vi "Autonomous Independent.vi"   [LabVIEW 2017]
doc: "This VI is called when autonomous begins, and will automatically be terminated when autonomous ends. You can carry out timed or sensor driven robot movement independently without needing to return to the caller."
uses:
  Public/Documents/Cross The Road Electronics/Phoenix-LabVIEW/Motor Controller/Controls/CTRE_Phoenix_MotorControl_ControlMode.ctl
  <vilib>/Rock Robotics/WPI/Solenoid/WPI_SolenoidValue.ctl
  <vilib>/Rock Robotics/WPI/Utilities/WPI_GetSetVariantRefNum.vi
  <vilib>/Rock Robotics/Network Tables/NT Read String.vi
  <vilib>/Rock Robotics/Network Tables/NT Write Numeric Array.vi
  <vilib>/Rock Robotics/WPI/Ultrasonic/WPI_SonarSRF04DigitalRefNum Registry Get.vi
  Public/Documents/Cross The Road Electronics/Phoenix-LabVIEW/Motor Controller/Get/CTRE_Phoenix_MotorController_GetSelectedSensorData.vi
  <vilib>/Rock Robotics/WPI/Solenoid/WPI_SolenoidSetEnum.vi
  Sling_MN_01/Global 1.vi
panel:
  # "Be sure to right-click and choose Data Operations>>Make Current Value default if you want to save the array values with the VI"
types:
  T1 = typedef "CTRE_Phoenix_MotorControl_ControlMode.ctl" = u16
  T2 = typedef "WPI_JoystickDevRef.ctl" = cluster{"Device":T3}
  T3 = typedef "WPI_JoystickDeviceEnum.ctl" = enum16{"USB 0", "USB 1", "USB 2", "USB 3", "USB 4", "USB 5"}
  T4 = typedef "WPI_GyroDevRef.ctl" = cluster{"DevStatus":errorcluster, "Analog Channel":T5, "Gain (VoltsPerDegree/Second)":dbl, "Gyro Type":enum16{"Analog", "XRS450"}, "Handle":i32, "SPI Bus":T6, "Device Found":bool, "Sample Rate":dbl, "Calibrate On Open":bool, "Offset":dbl}
  T5 = typedef "FPGA_AIChannel.ctl" = enum8{"AI 0", "AI 1", "AI 2", "AI 3", "AI MXP 0", "AI MXP 1", "AI MXP 2", "AI MXP 3", "Invalid"}
  T6 = typedef "spi_bus.ctl" = enum16{"SPI On-Board, CS0", "SPI On-Board, CS1", "SPI On-Board, CS2", "SPI On-Board, CS3", "SPI MXP", "Invalid"}
  T7 = typedef "WPI_MotorControlDeviceRef.ctl" = cluster{"DeviceStatus":errorcluster, "Type":T8, "PWM":cluster{"PWM Channel":T9, "DeadBand":T10}, "CAN":cluster{"Device Number":u8, "SetOutput VI Ref":variant, "GetOutput VI Ref":variant, "Enable VI Ref":variant, "Disable VI Ref":variant, "Data":variant}, "Invert":bool, "DIO PWM":cluster{"PWM \"Enable\" Channel":T9, "DIOChannel":T11, "PWM Rate":dbl}}
  T8 = typedef "WPI_MotorControlType.ctl" = enum16{"PWM", "CAN", "DIO PWM"}
  T9 = typedef "FPGA_DIOPWMChannel.ctl" = enum8{"PWM 0", "PWM 1", "PWM 2", "PWM 3", "PWM 4", "PWM 5", "PWM 6", "PWM 7", "PWM 8", "PWM 9", "PWM MXP 0", "PWM MXP 1", "PWM MXP 2", "PWM MXP 3", "PWM MXP 4", "PWM MXP 5", "PWM MXP 6", "PWM MXP 7", "PWM MXP 8", "PWM MXP 9", "Invalid"}
  T10 = typedef "WPI_PWMDeadband.ctl" = cluster{"Name":string, "maxPositivePwm":i32, "minPositivePwm":i32, "centerPwm":i32, "maxNegativePwm":i32, "minNegativePwm":i32, "angularRange":u16}
  T11 = typedef "FPGA_DIOChannel.ctl" = enum8{"DIO 0", "DIO 1", "DIO 2", "DIO 3", "DIO 4", "DIO 5", "DIO 6", "DIO 7", "DIO 8", "DIO 9", "DIO MXP 0", "DIO MXP 1", "DIO MXP 2", "DIO MXP 3", "DIO MXP 4", "DIO MXP 5", "DIO MXP 6", "DIO MXP 7", "DIO MXP 8", "DIO MXP 9", "DIO MXP 10", "DIO MXP 11", "DIO MXP 12", "DIO MXP 13", "DIO MXP 14", "DIO MXP 15", "SPI Port CS1", "SPI Port CS2", "SPI Port CS3", "SPI Port MISO", "SPI Port MOSI", "Invalid"}
  T12 = typedef "WPI_UltrasonicDeviceRef.ctl" = cluster{"DevStatus":errorcluster, "Ping Channel":T11, "Echo Channel":T11, "CntIndex":T13}
  T13 = typedef "FPGA_CounterCtrSystemIndex.ctl" = enum8{"Ctr 0", "Ctr 1", "Ctr 2", "Ctr 3", "Ctr 4", "Ctr 5", "Ctr 6", "Ctr 7", "Invalid"}
  T14 = typedef "WPI_SolenoidDevRef.ctl" = cluster{"DevStatus":errorcluster, "Pneumatics Control Module":u8, "Forward Solenoid Channel":T15, "Reverse Solenoid Channel":T15}
  T15 = typedef "WPI_SolenoidChannel.ctl" = enum8{"Solenoid 0", "Solenoid 1", "Solenoid 2", "Solenoid 3", "Solenoid 4", "Solenoid 5", "Solenoid 6", "Solenoid 7", "Invalid"}
  T16 = typedef "WPI_SolenoidValue.ctl" = enum16{"Off", "On", "Forward", "Reverse"}
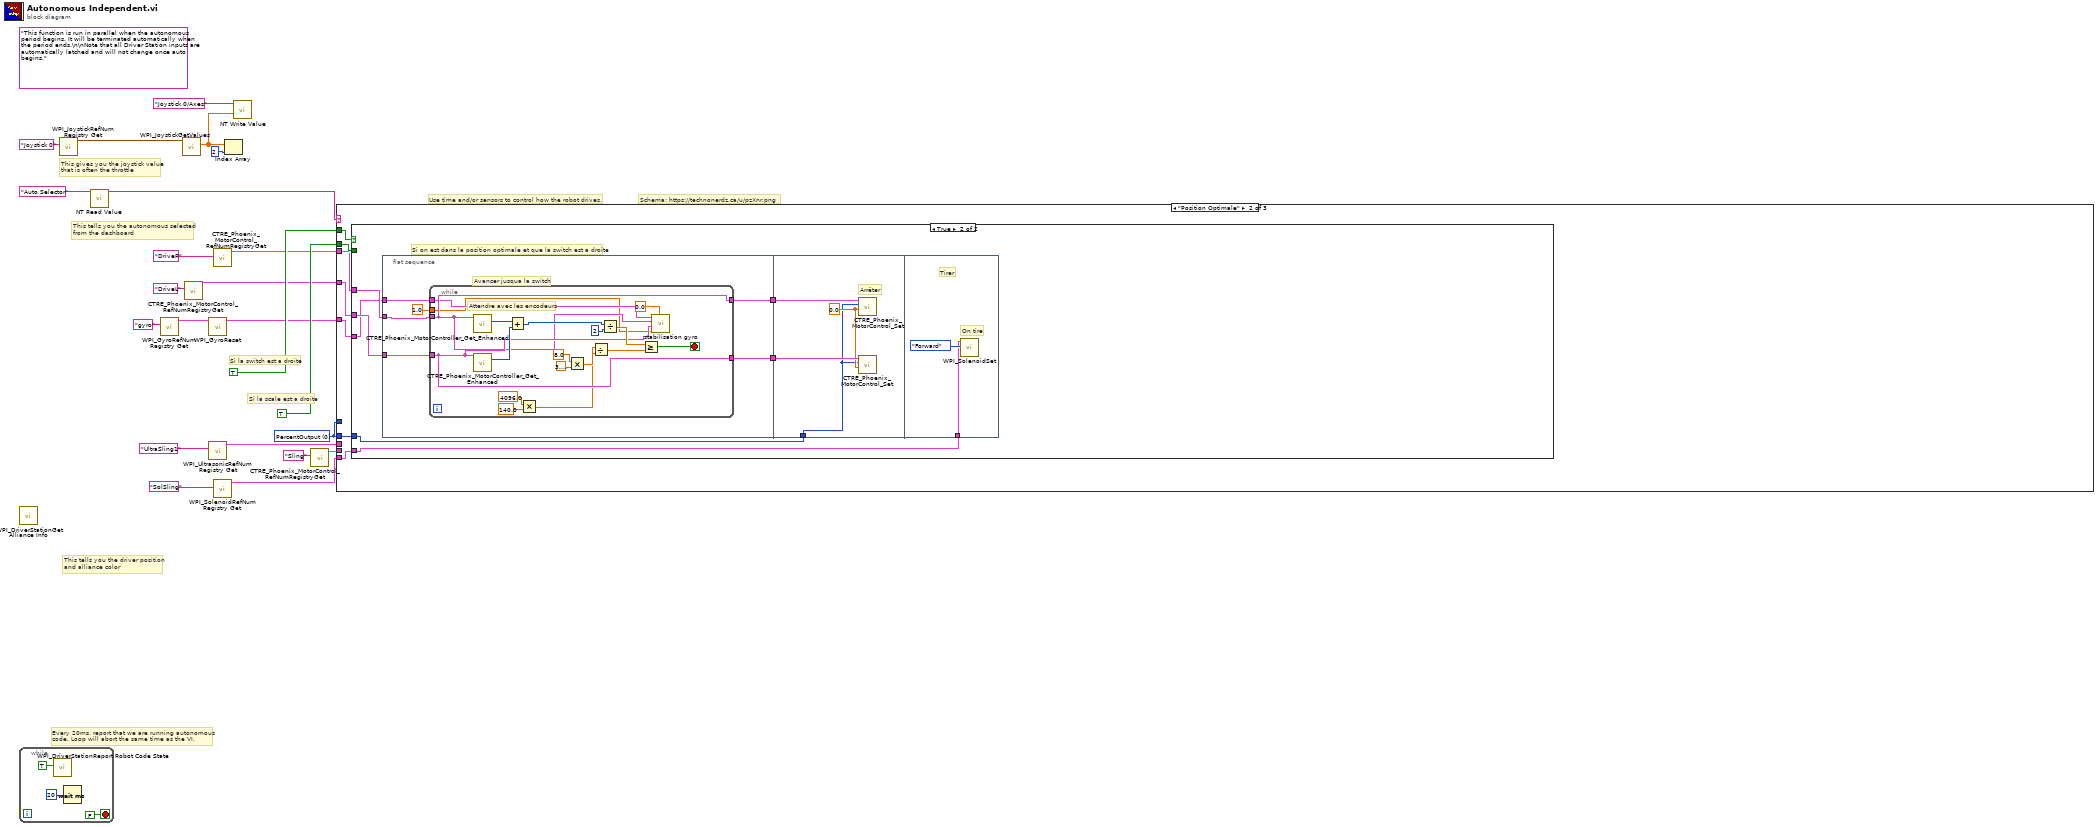
[diagram p0: block diagram]
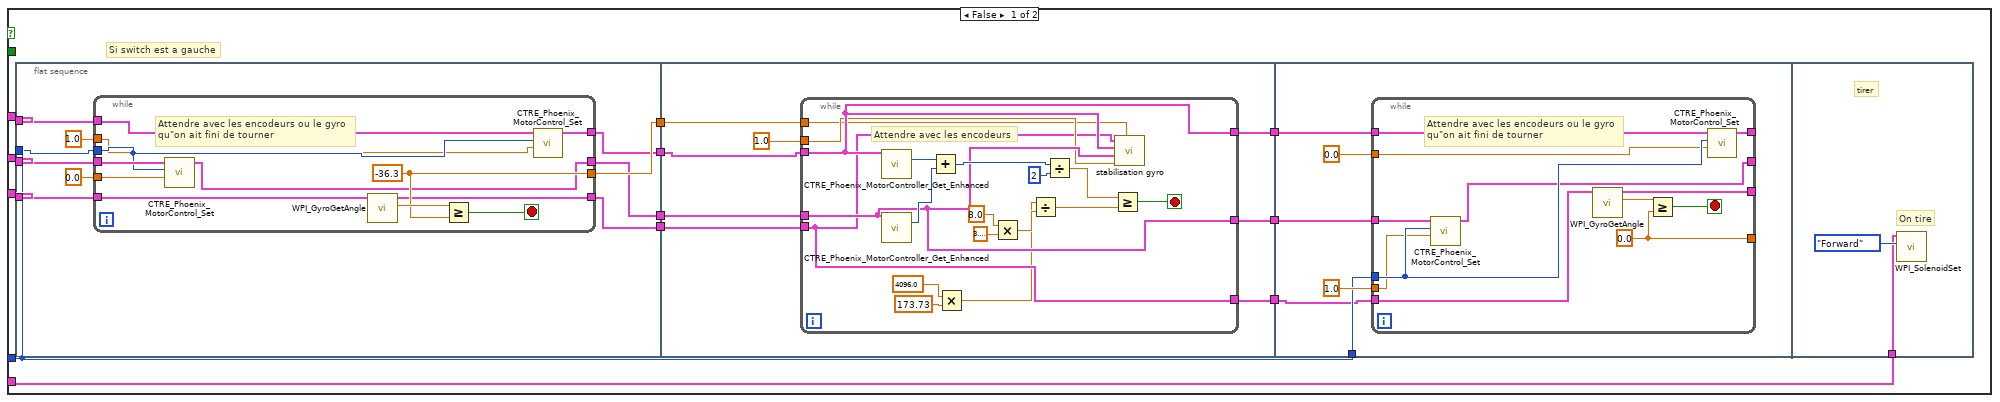
[diagram p3: hidden frame]
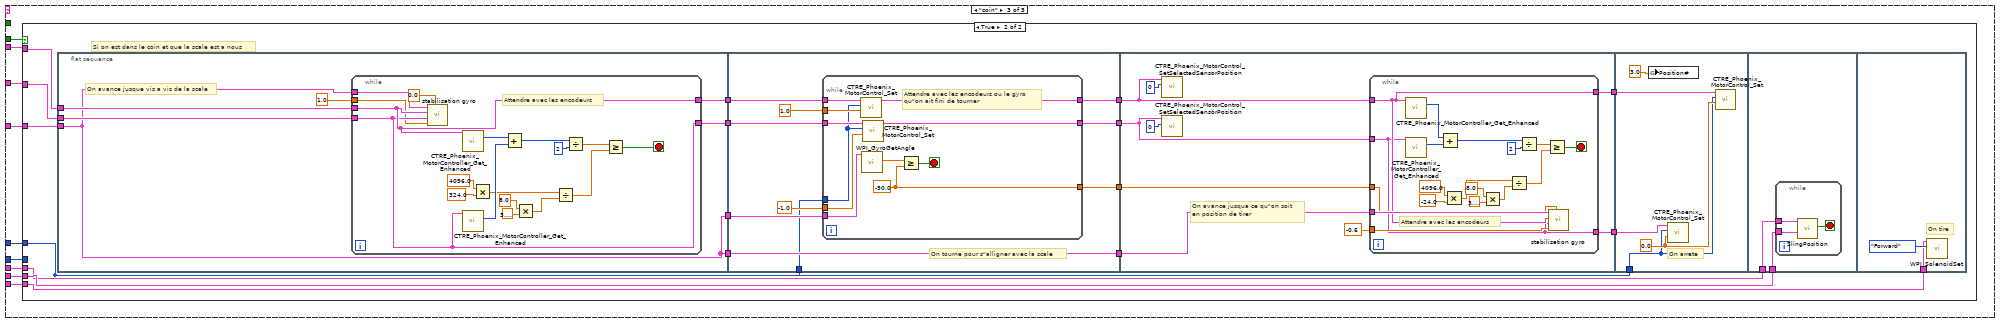
[diagram p4: hidden frame]
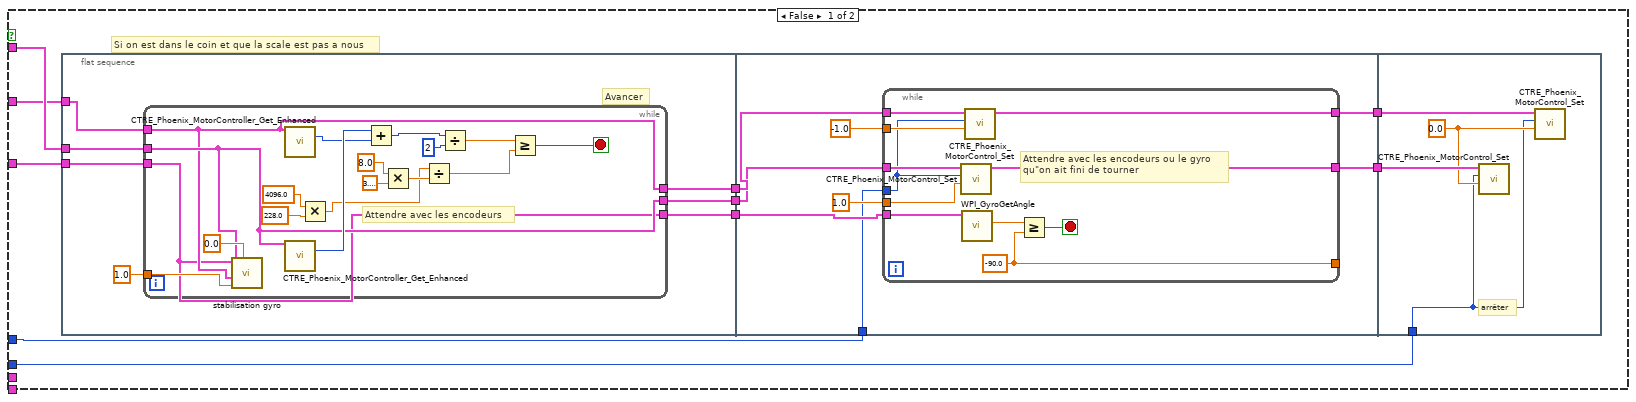
[diagram p5: hidden frame]
diagram:
  w7 = T1 0 items=["PercentOutput"=0, "Position"=1, "Velocity"=2, "Current"=3, "Follower"=5, "MotionProfile"=6, "MotionMagic"=7, "MotionMagicArc"=8, "MotionProfileArc"=10, "Disabled"=15] ("Control Mode")
  (unwired) "This function is run in parallel when the autonomous period begins. It will be terminated automatically when the period ends.\n\nNote that all Driver Station inputs are automatically latched and will not change once auto begins."
  # "Schema: https://technonerdz.ca/u/pzXnr.png"
  # "Si la switch est a droite"
  # "Si la scale est a droite"
  # "This tells you the autonomous selected\nfrom the dashboard"
  # "Every 20ms, report that we are running autonomous\ncode. Loop will abort the same time as the VI."
  # "This gives you the joystick value\nthat is often the throttle"
  # "Use time and/or sensors to control how the robot drives."
  # "This tells you the driver position\nand alliance color"
  n1 = call <vilib>:"WPI_DriverStationGet Alliance Info.vi"() -> ()  [unwired: 12 out]
  n2 = while {
    stop <- FALSE stop-if-true
    n3 = call <vilib>:"WPI_DriverStationReport Robot Code State.vi"("Autonomous"=TRUE) -> ()  [unwired: 10 in, 1 out]
    n4 = Wait (ms)(milliseconds to wait=u32 20) -> ()  [unwired: 1 out]
  }
  n5 = call <vilib>:"WPI_JoystickRefNum Registry Get.vi"("refnum name"="Joystick 0") -> ("JoystickDevRef"=w22:T2)  [unwired: 1 in, 9 out]
  n6 = call-poly <vilib>:"NT Read Value.vi"("Name"="Auto Selector") -> ("String"=w19:string)  [unwired: 9 in, 1 out]
  n7 = call <vilib>:"WPI_GyroRefNum Registry Get.vi"("refnum name"="gyro") -> ("GyroDevRef"=w9:T4)  [unwired: 9 in, 1 out]
  n8 = call <vilib>:"WPI_JoystickGetValues.vi"("JoystickDevRef"=w22) -> ("Axes"=w18:dbl[])  [unwired: 6 in, 4 out]
  n9 = call "CTRE_Phoenix_MotorControl_RefNumRegistryGet.vi"("refnum name"="DriveL") -> ("PhoenixMotorControlDevRef"=w11:T7)  [unwired: 9 in, 1 out]
  n10 = call <vilib>:"WPI_GyroReset.vi"("GyroDevRef"=w9) -> ("GyroDevRef"=w8:T4)  [unwired: 9 in, 1 out]
  n11 = call-poly <vilib>:"WPI_UltrasonicRefNum Registry Get.vi"("refnum name"="UltraSling1") -> ("SonarSRF04DevRef"=w1:T12)  [unwired: 9 in, 1 out]
  n12 = call "CTRE_Phoenix_MotorControl_RefNumRegistryGet.vi"("refnum name"="DriveR") -> ("PhoenixMotorControlDevRef"=w12:T7)  [unwired: 9 in, 1 out]
  n13 = call <vilib>:"WPI_SolenoidRefNum Registry Get.vi"("refnum name"="SolSling") -> ("SolenoidDevRef"=w5:T14)  [unwired: 9 in, 1 out]
  n14 = Index Array(array=w18, index=2) -> ()  [unwired: 1 out]
  n15 = call-poly <vilib>:"NT Write Value.vi"("Numeric Array"=w18, "Name"="Joystick 0/Axes") -> ()  [unwired: 9 in, 1 out]
  n16 = call "CTRE_Phoenix_MotorControl_RefNumRegistryGet.vi"("refnum name"="Sling") -> ("PhoenixMotorControlDevRef"=w2:T7)  [unwired: 9 in, 1 out]
  n17 = case shown="\"Position Optimale\"" w19 {
    tunnel: TRUE -> [_ w32 w159]
    tunnel: TRUE -> [_ w33 _]
    tunnel: w12 -> [_ w31 w158]
    tunnel: w11 -> [_ w30 w157]
    tunnel: w8 -> [_ w29 w156]
    tunnel: w7 -> [_ _ w155]
    tunnel: w7 -> [_ w28 w154]
    tunnel: w5 -> [_ w27 w153]
    tunnel: w2 -> [_ _ w152]
    tunnel: w1 -> [_ _ w151]
    frame Default {
      # "You can put your main auto here, or you can right-click on the case and make any\nother frame be the default case."
      # "This is the frame that will execute if no selection is made, or if it is not recognized"
    }
    frame "Position Optimale" {
      n18 = case shown="True" w33 {
        tunnel: w32 -> [_ _]
        tunnel: w31 -> [w45 w120]
        tunnel: w30 -> [w44 w119]
        tunnel: w29 -> [w43 w116]
        tunnel: w28 -> [w38 w115]
        tunnel: w27 -> [w34 w114]
        frame False {
          # "Si switch est a gauche"
          n19 = flat-sequence {
            tunnel: w45 -> [w55]
            tunnel: w44 -> [w54]
            tunnel: w38 -> [w53]
            tunnel: w43 -> [w50]
            tunnel: [w49] -> w42
            tunnel: [w48] -> w41
            tunnel: [w47] -> w40
            tunnel: [w46] -> w39
            tunnel: w42 -> [w74]
            tunnel: w41 -> [w73]
            tunnel: w40 -> [w72]
            tunnel: w39 -> [w71]
            tunnel: [w70] -> w37
            tunnel: [w69] -> w36
            tunnel: [w68] -> w35
            tunnel: w38 -> [w97]
            tunnel: w37 -> [w96]
            tunnel: w36 -> [w95]
            tunnel: w35 -> [w94]
            tunnel: w34 -> [w112]
            frame #0 {
              n20 = while {
                tunnel: w55 -> [w66]
                tunnel: w54 -> [w65]
                tunnel: w53 -> [w64]
                tunnel: 1.0 ("right") -> [w63]
                tunnel: 0.0 ("left") -> [w62]
                tunnel: w50 -> [w61]
                tunnel: [w59] -> w49
                tunnel: [w58] -> w48
                tunnel: [w57] -> w47
                tunnel: [w56] -> w46
                stop <- w60 stop-if-true
                w59 = -36.3 ("y")
                # "Attendre avec les encodeurs ou le gyro\nqu\"on ait fini de tourner"
                n21 = call "CTRE_Phoenix_MotorControl_Set.vi"("Output"=w62, "Control Mode"=w64, "PhoenixMotorControlDevRef"=w65) -> ("PhoenixMotorControlDevRef"=w58:T7)  [unwired: 7 in, 1 out]
                n22 = call <vilib>:"WPI_GyroGetAngle.vi"("GyroDevRef"=w61) -> ("Angle"=w67:dbl, "GyroDevRef"=w56:T4)  [unwired: 6 in, 3 out]
                n23 = Greater Or Equal?(x=w67, y=w59) -> (x >= y?=w60:bool)
                n24 = call "CTRE_Phoenix_MotorControl_Set.vi"("Output"=w63, "Control Mode"=w64, "PhoenixMotorControlDevRef"=w66) -> ("PhoenixMotorControlDevRef"=w57:T7)  [unwired: 7 in, 1 out]
              }
            }
            frame #1 {
              n25 = while {
                tunnel: 1.0 ("right") -> [w85]
                tunnel: w72 -> [w87]
                tunnel: w73 -> [w86]
                tunnel: [w87] -> w70
                tunnel: [w86] -> w69
                tunnel: [w83] -> w68
                tunnel: w74 -> [w84]
                tunnel: w71 -> [w83]
                stop <- w88 stop-if-true
                # "Attendre avec les encodeurs"
                n26 = call-poly "CTRE_Phoenix_MotorController_Get_Enhanced.vi"("PhoenixMotorControlDevRef"=w87) -> ("Position (Raw Sensor Units)"=w93:i32)  [unwired: 11 in, 3 out]
                n27 = call-poly "CTRE_Phoenix_MotorController_Get_Enhanced.vi"("PhoenixMotorControlDevRef"=w86) -> ("Position (Raw Sensor Units)"=w92:i32)  [unwired: 11 in, 3 out]
                n28 = Add(x=w93, y=w92) -> (x+y=w91:i32)
                n29 = Multiply(x=4096.0, y=173.73) -> (x*y=w81:dbl)
                n30 = Multiply(x=8.0, y=3.141592653589793) -> (x*y=w82:dbl)
                n31 = Divide(x=w81, y=w82) -> (x/y=w76:dbl)
                n32 = Divide(x=w91, y=2) -> (x/y=w89:dbl)
                n33 = Greater Or Equal?(x=w89, y=w76) -> (x >= y?=w88:bool)
                n34 = call "stabilisation gyro.vi"("Direction degres"=w84, "speed"=w85, "LeftMotorDevRef"=w86, "RightMotorDevRef"=w87, "gyroDevRef"=w83) -> ()  [unwired: 7 in]
              }
            }
            frame #2 {
              n35 = while {
                tunnel: w96 -> [w110]
                tunnel: w95 -> [w109]
                tunnel: w97 -> [w108]
                tunnel: 0.0 ("right") -> [w107]
                tunnel: 1.0 ("left") -> [w106]
                tunnel: w94 -> [w105]
                tunnel: [w103] -> _
                tunnel: [w102] -> _
                tunnel: [w101] -> _
                tunnel: [w100] -> _
                stop <- w104 stop-if-true
                w103 = 0.0 ("y")
                # "Attendre avec les encodeurs ou le gyro\nqu\"on ait fini de tourner"
                n36 = call "CTRE_Phoenix_MotorControl_Set.vi"("Output"=w106, "Control Mode"=w108, "PhoenixMotorControlDevRef"=w109) -> ("PhoenixMotorControlDevRef"=w102:T7)  [unwired: 7 in, 1 out]
                n37 = call <vilib>:"WPI_GyroGetAngle.vi"("GyroDevRef"=w105) -> ("Angle"=w111:dbl, "GyroDevRef"=w100:T4)  [unwired: 6 in, 3 out]
                n38 = Greater Or Equal?(x=w111, y=w103) -> (x >= y?=w104:bool)
                n39 = call "CTRE_Phoenix_MotorControl_Set.vi"("Output"=w107, "Control Mode"=w108, "PhoenixMotorControlDevRef"=w110) -> ("PhoenixMotorControlDevRef"=w101:T7)  [unwired: 7 in, 1 out]
              }
            }
            frame #3 {
              # "On tire"
              # "tirer"
              n40 = call-poly <vilib>:"WPI_SolenoidSet.vi"("Value"=WPI_SolenoidValue."Forward", "SolenoidDevRef"=w112) -> ()  [unwired: 8 in, 2 out]
            }
          }
        }
        frame True {
          # "Si on est dans la position optimale et que la switch est a droite"
          n41 = flat-sequence {
            tunnel: w120 -> [w125]
            tunnel: w119 -> [w124]
            tunnel: [w123] -> w118
            tunnel: [w122] -> w117
            tunnel: w116 -> [w121]
            tunnel: w118 -> [w148]
            tunnel: w117 -> [w147]
            tunnel: w115 -> [w145]
            tunnel: w114 -> [w149]
            frame #0 {
              # "Avancer jusqua la switch"
              n42 = while {
                tunnel: 1.0 ("right") -> [w134]
                tunnel: w125 -> [w137]
                tunnel: w124 -> [w138]
                tunnel: [w138] -> w123
                tunnel: [w137] -> w122
                tunnel: w121 -> [w136]
                stop <- w139 stop-if-true
                # "Attendre avec les encodeurs"
                n43 = call-poly "CTRE_Phoenix_MotorController_Get_Enhanced.vi"("PhoenixMotorControlDevRef"=w137) -> ("Position (Raw Sensor Units)"=w144:i32)  [unwired: 11 in, 3 out]
                n44 = call-poly "CTRE_Phoenix_MotorController_Get_Enhanced.vi"("PhoenixMotorControlDevRef"=w138) -> ("Position (Raw Sensor Units)"=w143:i32)  [unwired: 11 in, 3 out]
                n45 = Add(x=w144, y=w143) -> (x+y=w142:i32)
                n46 = Multiply(x=4096.0, y=140.0) -> (x*y=w132:dbl)
                n47 = Multiply(x=8.0, y=3.141592653589793) -> (x*y=w133:dbl)
                n48 = Divide(x=w132, y=w133) -> (x/y=w127:dbl)
                n49 = Divide(x=w142, y=2) -> (x/y=w140:dbl)
                n50 = Greater Or Equal?(x=w140, y=w127) -> (x >= y?=w139:bool)
                n51 = call "stabilisation gyro.vi"("Direction degres"=0.0, "speed"=w134, "LeftMotorDevRef"=w138, "RightMotorDevRef"=w137, "gyroDevRef"=w136) -> ()  [unwired: 7 in]
              }
            }
            frame #1 {
              w146 = 0.0 ("Output")
              # "Arrêter"
              n52 = call "CTRE_Phoenix_MotorControl_Set.vi"("Output"=w146, "Control Mode"=w145, "PhoenixMotorControlDevRef"=w147) -> ()  [unwired: 7 in, 2 out]
              n53 = call "CTRE_Phoenix_MotorControl_Set.vi"("Output"=w146, "Control Mode"=w145, "PhoenixMotorControlDevRef"=w148) -> ()  [unwired: 7 in, 2 out]
            }
            frame #2 {
              # "On tire"
              # "Tirer"
              n54 = call-poly <vilib>:"WPI_SolenoidSet.vi"("Value"=WPI_SolenoidValue."Forward", "SolenoidDevRef"=w149) -> ()  [unwired: 8 in, 2 out]
            }
          }
        }
      }
    }
    frame "coin" {
      n55 = case shown="True" w159 {
        tunnel: w158 -> [w169 w234]
        tunnel: w157 -> [w168 w233]
        tunnel: w156 -> [w167 w226]
        tunnel: w155 -> [w160 w221]
        tunnel: w154 -> [w166 _]
        tunnel: w153 -> [_ w220]
        tunnel: w152 -> [_ w219]
        tunnel: w151 -> [_ w218]
        frame False {
          # "Si on est dans le coin et que la scale est pas a nous"
          n56 = flat-sequence {
            tunnel: w169 -> [w175]
            tunnel: w168 -> [w174]
            tunnel: [w173] -> w165
            tunnel: [w172] -> w163
            tunnel: w167 -> [w171]
            tunnel: [w170] -> w161
            tunnel: w165 -> [w198]
            tunnel: [w196] -> w164
            tunnel: w163 -> [w199]
            tunnel: [w197] -> w162
            tunnel: w161 -> [w200]
            tunnel: w160 -> [w195]
            tunnel: w164 -> [w217]
            tunnel: w162 -> [w216]
            tunnel: w166 -> [w214]
            frame #0 {
              # "Avancer"
              n57 = while {
                tunnel: 1.0 ("right") -> [w185]
                tunnel: w175 -> [w187]
                tunnel: w174 -> [w186]
                tunnel: [w187] -> w173
                tunnel: [w186] -> w172
                tunnel: w171 -> [w177]
                tunnel: [w177] -> w170
                stop <- w189 stop-if-true
                # "Attendre avec les encodeurs"
                n58 = call "stabilisation gyro.vi"("Direction degres"=0.0, "speed"=w185, "LeftMotorDevRef"=w186, "RightMotorDevRef"=w187, "gyroDevRef"=w177) -> ()  [unwired: 7 in]
                n59 = call-poly "CTRE_Phoenix_MotorController_Get_Enhanced.vi"("PhoenixMotorControlDevRef"=w186) -> ("Position (Raw Sensor Units)"=w193:i32)  [unwired: 11 in, 3 out]
                n60 = call-poly "CTRE_Phoenix_MotorController_Get_Enhanced.vi"("PhoenixMotorControlDevRef"=w187) -> ("Position (Raw Sensor Units)"=w194:i32)  [unwired: 11 in, 3 out]
                n61 = Multiply(x=4096.0, y=228.0) -> (x*y=w183:dbl)
                n62 = Add(x=w194, y=w193) -> (x+y=w192:i32)
                n63 = Multiply(x=8.0, y=3.141592653589793) -> (x*y=w184:dbl)
                n64 = Divide(x=w183, y=w184) -> (x/y=w178:dbl)
                n65 = Divide(x=w192, y=2) -> (x/y=w190:dbl)
                n66 = Greater Or Equal?(x=w190, y=w178) -> (x >= y?=w189:bool)
              }
            }
            frame #1 {
              n67 = while {
                tunnel: -1.0 ("left") -> [w211]
                tunnel: 1.0 ("right") -> [w212]
                tunnel: w198 -> [w213]
                tunnel: w199 -> [w210]
                tunnel: [w209] -> w196
                tunnel: [w208] -> w197
                tunnel: w200 -> [w205]
                tunnel: [w204] -> _
                tunnel: w195 -> [w203]
                stop <- w206 stop-if-true
                w204 = -90.0 ("y")
                # "Attendre avec les encodeurs ou le gyro\nqu\"on ait fini de tourner"
                n68 = call "CTRE_Phoenix_MotorControl_Set.vi"("Output"=w212, "Control Mode"=w203, "PhoenixMotorControlDevRef"=w213) -> ("PhoenixMotorControlDevRef"=w209:T7)  [unwired: 7 in, 1 out]
                n69 = call <vilib>:"WPI_GyroGetAngle.vi"("GyroDevRef"=w205) -> ("Angle"=w207:dbl)  [unwired: 6 in, 4 out]
                n70 = call "CTRE_Phoenix_MotorControl_Set.vi"("Output"=w211, "Control Mode"=w203, "PhoenixMotorControlDevRef"=w210) -> ("PhoenixMotorControlDevRef"=w208:T7)  [unwired: 7 in, 1 out]
                n71 = Greater Or Equal?(x=w207, y=w204) -> (x >= y?=w206:bool)
              }
            }
            frame #2 {
              w215 = 0.0 ("Output")
              # "arrêter"
              n72 = call "CTRE_Phoenix_MotorControl_Set.vi"("Output"=w215, "Control Mode"=w214, "PhoenixMotorControlDevRef"=w217) -> ()  [unwired: 7 in, 2 out]
              n73 = call "CTRE_Phoenix_MotorControl_Set.vi"("Output"=w215, "Control Mode"=w214, "PhoenixMotorControlDevRef"=w216) -> ()  [unwired: 7 in, 2 out]
            }
          }
        }
        frame True {
          # "Si on est dans le coin et que la scale est a nous"
          n74 = flat-sequence {
            tunnel: [w237] -> w232
            tunnel: [w236] -> w231
            tunnel: [w235] -> w225
            tunnel: [w235] -> w224
            tunnel: w234 -> [w239]
            tunnel: w233 -> [w238]
            tunnel: w226 -> [w235]
            tunnel: w232 -> [w266]
            tunnel: w231 -> [w265]
            tunnel: [w264] -> w230
            tunnel: [w263] -> w229
            tunnel: w225 -> [w262]
            tunnel: w224 -> [w261]
            tunnel: [w261] -> w223
            tunnel: [w260] -> w222
            tunnel: w221 -> [w259]
            tunnel: w230 -> [w281]
            tunnel: w229 -> [w287]
            tunnel: [w286] -> w228
            tunnel: [w285] -> w227
            tunnel: w223 -> [w284]
            tunnel: w222 -> [w283]
            tunnel: w228 -> [w311]
            tunnel: w227 -> [w310]
            tunnel: w221 -> [w308]
            tunnel: w219 -> [w313]
            tunnel: w218 -> [w312]
            tunnel: w220 -> [w317]
            frame #0 {
              # "On avance jusque vis a vis de la scale"
              n75 = while {
                tunnel: 1.0 ("right") -> [w249]
                tunnel: w239 -> [w251]
                tunnel: w238 -> [w250]
                tunnel: [w251] -> w237
                tunnel: [w250] -> w236
                tunnel: w235 -> [w252]
                stop <- w253 stop-if-true
                # "Attendre avec les encodeurs"
                n76 = call "stabilisation gyro.vi"("Direction degres"=0.0, "speed"=w249, "LeftMotorDevRef"=w250, "RightMotorDevRef"=w251, "gyroDevRef"=w252) -> ()  [unwired: 7 in]
                n77 = call-poly "CTRE_Phoenix_MotorController_Get_Enhanced.vi"("PhoenixMotorControlDevRef"=w251) -> ("Position (Raw Sensor Units)"=w258:i32)  [unwired: 11 in, 3 out]
                n78 = call-poly "CTRE_Phoenix_MotorController_Get_Enhanced.vi"("PhoenixMotorControlDevRef"=w250) -> ("Position (Raw Sensor Units)"=w257:i32)  [unwired: 11 in, 3 out]
                n79 = Multiply(x=4096.0, y=324.0) -> (x*y=w246:dbl)
                n80 = Add(x=w258, y=w257) -> (x+y=w256:i32)
                n81 = Multiply(x=8.0, y=3.141592653589793) -> (x*y=w247:dbl)
                n82 = Divide(x=w246, y=w247) -> (x/y=w241:dbl)
                n83 = Divide(x=w256, y=2) -> (x/y=w254:dbl)
                n84 = Greater Or Equal?(x=w254, y=w241) -> (x >= y?=w253:bool)
              }
            }
            frame #1 {
              # "On tourne pour s\"alligner avec la scale"
              n85 = while {
                tunnel: -1.0 ("left") -> [w277]
                tunnel: 1.0 ("right") -> [w278]
                tunnel: w266 -> [w279]
                tunnel: w265 -> [w276]
                tunnel: [w275] -> w264
                tunnel: [w274] -> w263
                tunnel: w262 -> [w271]
                tunnel: [w270] -> w260
                tunnel: w259 -> [w269]
                stop <- w272 stop-if-true
                w270 = -90.0 ("y")
                # "Attendre avec les encodeurs ou le gyro\nqu\"on ait fini de tourner"
                n86 = call "CTRE_Phoenix_MotorControl_Set.vi"("Output"=w278, "Control Mode"=w269, "PhoenixMotorControlDevRef"=w279) -> ("PhoenixMotorControlDevRef"=w275:T7)  [unwired: 7 in, 1 out]
                n87 = call <vilib>:"WPI_GyroGetAngle.vi"("GyroDevRef"=w271) -> ("Angle"=w273:dbl)  [unwired: 6 in, 4 out]
                n88 = call "CTRE_Phoenix_MotorControl_Set.vi"("Output"=w277, "Control Mode"=w269, "PhoenixMotorControlDevRef"=w276) -> ("PhoenixMotorControlDevRef"=w274:T7)  [unwired: 7 in, 1 out]
                n89 = Greater Or Equal?(x=w273, y=w270) -> (x >= y?=w272:bool)
              }
            }
            frame #2 {
              # "On avance jusqua ce qu\"on soit\nen position de tirer"
              n90 = call <vilib>:"CTRE_Phoenix_MotorControl_SetSelectedSensorPosition.vi"("New Sensor Position"=0, "PhoenixMotorControlDevRef"=w281) -> ()  [unwired: 8 in, 2 out]
              n91 = call <vilib>:"CTRE_Phoenix_MotorControl_SetSelectedSensorPosition.vi"("New Sensor Position"=0, "PhoenixMotorControlDevRef"=w287) -> ()  [unwired: 8 in, 2 out]
              n92 = while {
                tunnel: -0.6 ("right") -> [w300]
                tunnel: w281 -> [w298]
                tunnel: w287 -> [w289]
                tunnel: [w298] -> w286
                tunnel: [w289] -> w285
                tunnel: w284 -> [w299]
                tunnel: w283 -> [w297]
                stop <- w301 stop-if-true
                # "Attendre avec les encodeurs"
                n93 = call-poly "CTRE_Phoenix_MotorController_Get_Enhanced.vi"("PhoenixMotorControlDevRef"=w298) -> ("Position (Raw Sensor Units)"=w306:i32)  [unwired: 11 in, 3 out]
                n94 = call-poly "CTRE_Phoenix_MotorController_Get_Enhanced.vi"("PhoenixMotorControlDevRef"=w289) -> ("Position (Raw Sensor Units)"=w305:i32)  [unwired: 11 in, 3 out]
                n95 = Add(x=w306, y=w305) -> (x+y=w304:i32)
                n96 = Multiply(x=4096.0, y=-24.0) -> (x*y=w295:dbl)
                n97 = Multiply(x=8.0, y=3.141592653589793) -> (x*y=w296:dbl)
                n98 = Divide(x=w295, y=w296) -> (x/y=w290:dbl)
                n99 = Divide(x=w304, y=2) -> (x/y=w302:dbl)
                n100 = Greater Or Equal?(x=w302, y=w290) -> (x >= y?=w301:bool)
                n101 = call "stabilisation gyro.vi"("Direction degres"=w297, "speed"=w300, "LeftMotorDevRef"=w289, "RightMotorDevRef"=w298, "gyroDevRef"=w299) -> ()  [unwired: 7 in]
              }
            }
            frame #3 {
              w309 = 0.0 ("Output")
              # "On arrete"
              n102 = global write "Global 1.vi" "Position#"(3.0 ("Position#")) -> ()
              n103 = call "CTRE_Phoenix_MotorControl_Set.vi"("Output"=w309, "Control Mode"=w308, "PhoenixMotorControlDevRef"=w310) -> ()  [unwired: 7 in, 2 out]
              n104 = call "CTRE_Phoenix_MotorControl_Set.vi"("Output"=w309, "Control Mode"=w308, "PhoenixMotorControlDevRef"=w311) -> ()  [unwired: 7 in, 2 out]
            }
            frame #4 {
              n105 = while {
                tunnel: w313 -> [w316]
                tunnel: w312 -> [w315]
                stop <- w314 stop-if-true
                n106 = call "SlingPosition.vi"("PhoenixMotorControlDevRef"=w316, "SonarSRF04DevRef"=w315) -> ("Ready"=w314:bool)  [unwired: 9 in]
              }
            }
            frame #5 {
              # "On tire"
              n107 = call-poly <vilib>:"WPI_SolenoidSet.vi"("Value"=WPI_SolenoidValue."Forward", "SolenoidDevRef"=w317) -> ()  [unwired: 8 in, 2 out]
            }
          }
        }
      }
    }
  }
